vi "Prepare Config.vi"(8 "Error In":errorcluster, 11 "FileConfig In":refnum<class "FileConfig.lvclass">) -> (0 "Error Out":errorcluster, 3 "FileConfig Out":refnum<class "FileConfig.lvclass">)   [LabVIEW 2020, in "FileConfig.lvclass"]
uses:
  FileConfig.lvclass
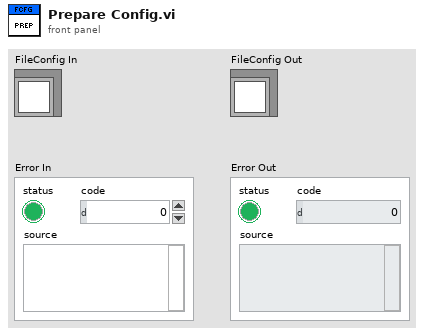
[diagram p1: front panel]
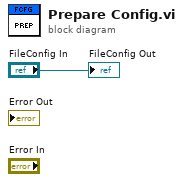
[diagram p0: block diagram]
diagram:
  "FileConfig Out" <- "FileConfig In"
